vi "Get MathFunction Name.vi"(8 "error in (no error)":errorcluster, 11 "Subtract in":refnum<class "Subtract.lvclass">) -> (0 "error out":errorcluster, 2 "MathFunction Name":string, 3 "Subtract out":refnum<class "Subtract.lvclass">)   [LabVIEW 2019, in "lv-classprovidershell-example.lvlib" / "Subtract.lvclass"]
uses:
  Subtract.lvclass
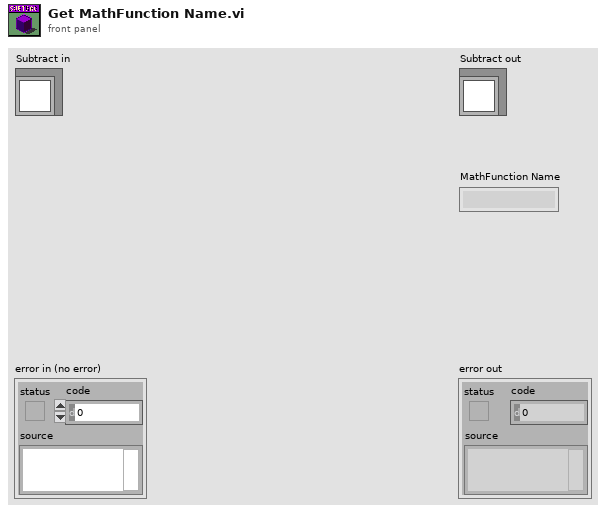
[diagram p1: front panel]
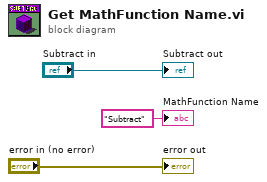
[diagram p0: block diagram]
diagram:
  "error out" <- "error in (no error)"
  "Subtract out" <- "Subtract in"
  "MathFunction Name" <- "Subtract" ("MathFunction Name")
